vi "Reasons For Termination.vi"(11 "Reason for last heating cycle termination":u16) -> (3 "String":string)   [LabVIEW 2023]
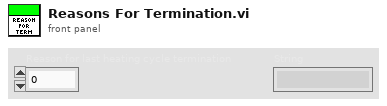
[diagram p1: front panel]
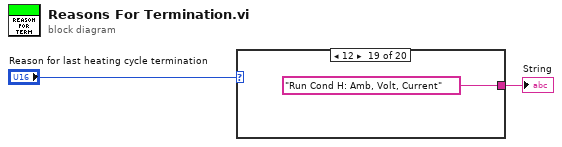
[diagram p0: block diagram]
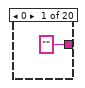
[diagram p2: hidden frame]
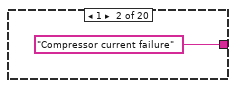
[diagram p3: hidden frame]
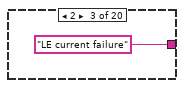
[diagram p4: hidden frame]
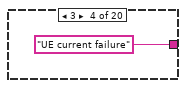
[diagram p5: hidden frame]
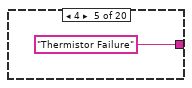
[diagram p6: hidden frame]
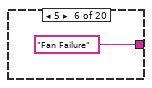
[diagram p7: hidden frame]
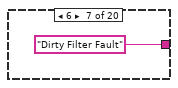
[diagram p8: hidden frame]
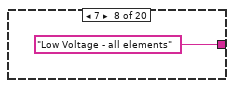
[diagram p9: hidden frame]
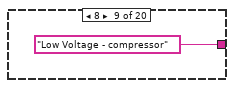
[diagram p10: hidden frame]
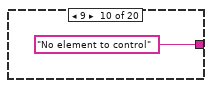
[diagram p11: hidden frame]
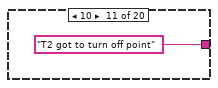
[diagram p12: hidden frame]
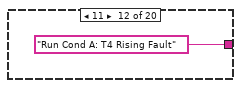
[diagram p13: hidden frame]
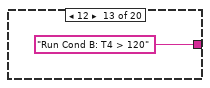
[diagram p14: hidden frame]
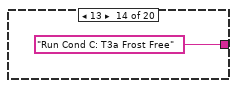
[diagram p15: hidden frame]
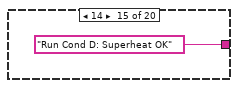
[diagram p16: hidden frame]
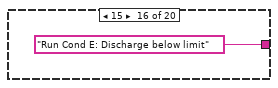
[diagram p17: hidden frame]
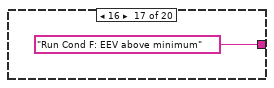
[diagram p18: hidden frame]
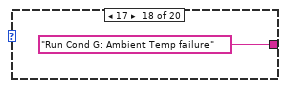
[diagram p19: hidden frame]
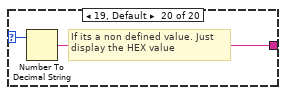
[diagram p20: hidden frame]
diagram:
  n1 = case shown="12" "Reason for last heating cycle termination" {
    selector: "Reason for last heating cycle termination" -> [_ _ _ _ _ _ _ _ _ _ _ _ _ _ _ _ _ _ _ w23]
    tunnel: ["" "Compressor current failure" "LE current failure" "UE current failure" "Thermistor Failure" "Fan Failure" "Dirty Filter Fault" "Low Voltage - all elements" "Low Voltage - compressor" "No element to control" "T2 got to turn off point" "Run Cond A: T4 Rising Fault" "Run Cond B: T4 > 120" "Run Cond C: T3a Frost Free" "Run Cond D: Superheat OK" "Run Cond E: Discharge below limit" "Run Cond F: EEV above minimum" "Run Cond G: Ambient Temp failure" "Run Cond H: Amb, Volt, Current" w22] -> w2
    frame 0 {
    }
    frame 1 {
    }
    frame 2 {
    }
    frame 3 {
    }
    frame 4 {
    }
    frame 5 {
    }
    frame 6 {
    }
    frame 7 {
    }
    frame 8 {
    }
    frame 9 {
    }
    frame 10 {
    }
    frame 11 {
    }
    frame 12 {
    }
    frame 13 {
    }
    frame 14 {
    }
    frame 15 {
    }
    frame 16 {
    }
    frame 17 {
    }
    frame 18 {
    }
    frame 19, Default {
      # "If its a non defined value. Just \ndisplay the HEX value"
      n2 = Number To Decimal String(number=w23) -> (decimal integer string=w22:string)  [unwired: 1 in]
    }
  }
  "String" <- w2
